vi "Handle Message.vi"(5 "Stack ID":u8, 7 "Function ID":u8, 8 "error in (no error)":errorcluster, 10 "Data":string, 11 "Template in":refnum<class "Template.lvclass">) -> (0 "error out":errorcluster, 1 "Send Answer":bool, 2 "Answer":variant, 3 "Template out":refnum<class "Template.lvclass">)   [LabVIEW 2011, in "Tinkerforge.lvlib" / "Template.lvclass"]
doc: "This VI is the child implementation of \"Handle Message.vi\" and processes all responses for this device type."
uses:
  Template.lvclass
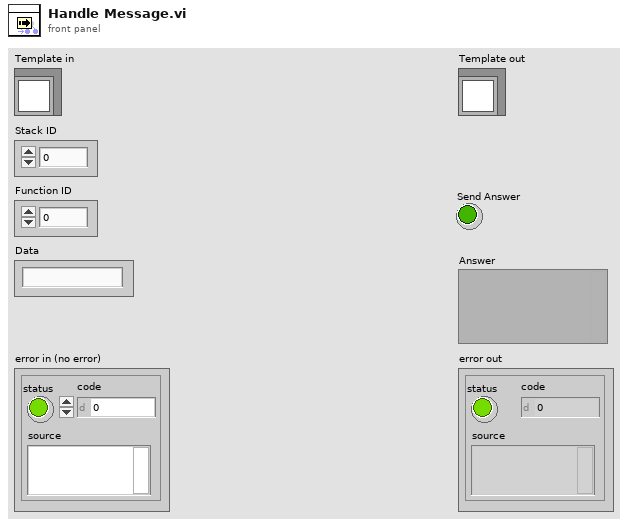
[diagram p1: front panel]
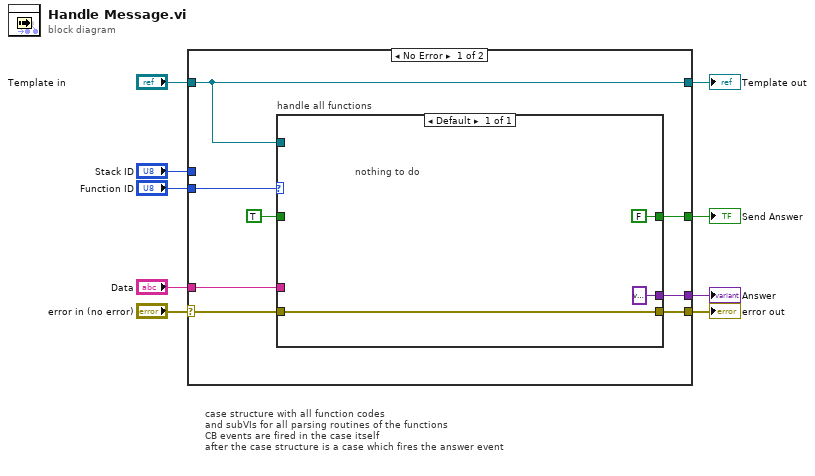
[diagram p0: block diagram]
diagram:
  # "case structure with all function codes\nand subVIs for all parsing routines of the functions\nCB events are fired in the case itself\nafter the case structure is a case which fires the answer event"
  n1 = case shown="No Error" "error in (no error)" {
    selector: "error in (no error)" -> [w14 w21]
    tunnel: "Template in" -> [w17 w22]
    tunnel: "Stack ID" -> [_ _]
    tunnel: "Function ID" -> [w16 _]
    tunnel: "Data" -> [w13 _]
    tunnel: [w17 w22] -> w4
    tunnel: [w12 w21] -> w3
    tunnel: [w11 _] -> w2
    tunnel: [w10 _] -> w1
    frame No Error {
      n2 = case "handle all functions" shown="Default" w16 {
        tunnel: w14 -> [w20]
        tunnel: TRUE -> [_]
        tunnel: [FALSE] -> w10
        tunnel: [w20] -> w12
        tunnel: [variant ("Variant")] -> w11
        tunnel: w17 -> [_]
        tunnel: w13 -> [_]
        frame Default {
          # "nothing to do"
        }
      }
    }
    frame Error {
    }
  }
  "error out" <- w3
  "Template out" <- w4
  "Answer" <- w2
  "Send Answer" <- w1
